vi "Delete Element at Beginning.vi"(8 "error in (no error)":errorcluster, 11 "Variant in":variant) -> (0 "error out":errorcluster, 1 "element":variant, 2 "Name":string, 3 "Variant out":variant)   [LabVIEW 2017, in "Advanced Variant Tools.lvlib" / "Cluster Manipulation.lvlib"]
uses:
  Cluster Manipulation.lvlib
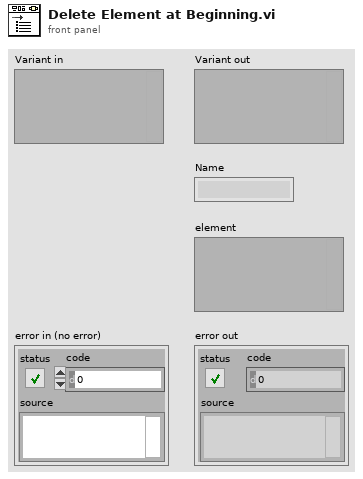
[diagram p1: front panel]
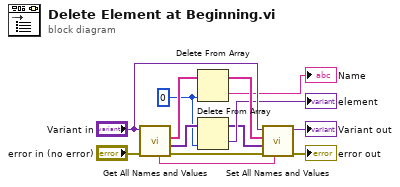
[diagram p0: block diagram]
diagram:
  w2 = 0 ("index")
  n1 = call "Get All Names and Values.vi"("error in"="error in (no error)", "Cluster In"="Variant in") -> ("error out"=w12:errorcluster, "Values"=w4:variant[], "Item Names"=w8:string[], "Name"=w1:string)  [unwired: 5 in, 1 out]
  n2 = Delete From Array(array=w8, index=w2) -> (deleted portion=→"Name":string, array with subset deleted=w7:string[])  [unwired: 1 in]
  n3 = Delete From Array(array=w4, index=w2) -> (deleted portion=→"element":variant, array with subset deleted=w3:variant[])  [unwired: 1 in]
  n4 = call "Set All Names and Values.vi"("Name"=w1, "error in"=w12, "values"=w3, "Item Names"=w7, "Cluster In"="Variant in") -> ("error out"=→"error out":errorcluster, "Cluster Out"=→"Variant out":variant)  [unwired: 5 in]
